vi "sequencerCore.vi"   [LabVIEW 2014]
uses:
  sequencerState.ctl
  Controls/heinzingerSelect.ctl
  <vilib>/rvi/Emulation/niFpgaGetClockAttributes.vi
  <vilib>/rvi/Emulation/niFpgaSctlEmulationGetInTimedLoop.vi
  <vilib>/rvi/Emulation/niFpgaEmulationReportErrorSimple.vi
  <vilib>/rvi/Emulation/niFpgaCriticalErrorInLSC.vi
types:
  T1 = typedef "sequencerState.ctl" = enum16{"init", "idle", "writeGlobVars", "measureOffset", "measureTrack", "measComplete", "error"}
  T2 = typedef "heinzingerSelect.ctl" = enum8{"Kepco", "Heinzinger0", "Heinzinger1", "Heinzinger2"}
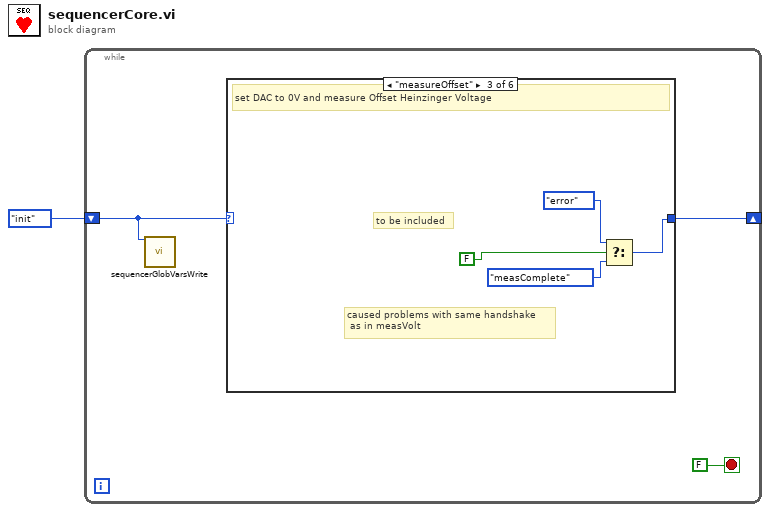
[diagram p0: block diagram]
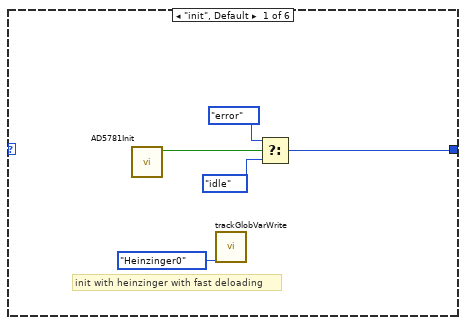
[diagram p2: hidden frame]
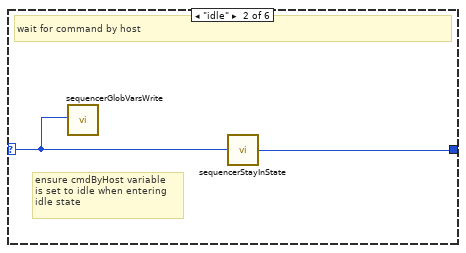
[diagram p3: hidden frame]
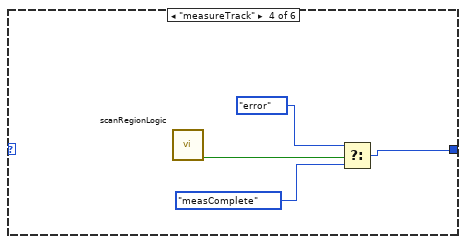
[diagram p4: hidden frame]
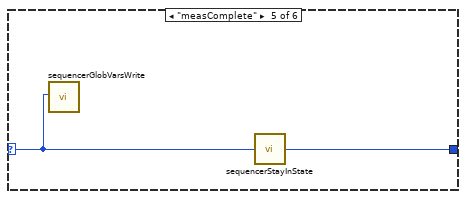
[diagram p5: hidden frame]
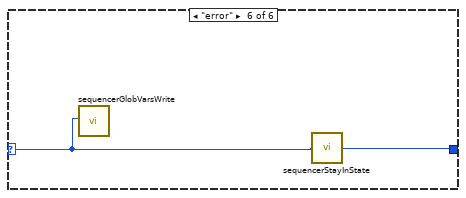
[diagram p6: hidden frame]
diagram:
  n1 = while {
    shift-right: [w2] -> _
    shift-left: sequencerState."init" ("Enum") -> [w3]
    stop <- FALSE stop-if-true
    n2 = call "sequencerGlobVarsWrite.vi"("fpgaState"=w3) -> ()  [unwired: 19 in]
    n3 = case shown="\"measureOffset\"" w3 {
      selector: w3 -> [_ w11 _ _ w21 w23]
      tunnel: [w6 w10 w15 w16 w20 w22] -> w2
      frame "init", Default {
        # "init with heinzinger with fast deloading"
        n4 = call "AD5781Init.vi"() -> ("timeOut"=w7:bool)  [unwired: 11 in]
        n5 = call "trackGlobVarWrite.vi"("heinzingerControl"=heinzingerSelect."Heinzinger0") -> ()  [unwired: 19 in]
        n6 = Select(t=sequencerState."error", s=w7, f=sequencerState."idle" ("Enum")) -> (s? t:f=w6:T1)
      }
      frame "idle" {
        # "ensure cmdByHost variable \nis set to idle when entering\nidle state"
        # "wait for command by host"
        n7 = call "sequencerGlobVarsWrite.vi"("cmdByHost"=w11) -> ()  [unwired: 19 in]
        n8 = call "sequencerStayInState.vi"("stateBefore"=w11) -> ("cmdByHost"=w10:T1)  [unwired: 4 in]
      }
      frame "measureOffset" {
        # "caused problems with same handshake\n as in measVolt"
        # "to be included"
        # "set DAC to 0V and measure Offset Heinzinger Voltage"
        n9 = Select(t=sequencerState."error" ("cmdFromHost"), s=FALSE, f=sequencerState."measComplete" ("cmdFromHost")) -> (s? t:f=w15:T1)
      }
      frame "measureTrack" {
        n10 = call "scanRegionLogic.vi"() -> ("Error"=w17:bool)  [unwired: 11 in]
        n11 = Select(t=sequencerState."error" ("Enum"), s=w17, f=sequencerState."measComplete" ("Enum")) -> (s? t:f=w16:T1)
      }
      frame "measComplete" {
        n12 = call "sequencerGlobVarsWrite.vi"("cmdByHost"=w21) -> ()  [unwired: 19 in]
        n13 = call "sequencerStayInState.vi"("stateBefore"=w21) -> ("cmdByHost"=w20:T1)  [unwired: 4 in]
      }
      frame "error" {
        n14 = call "sequencerGlobVarsWrite.vi"("cmdByHost"=w23) -> ()  [unwired: 19 in]
        n15 = call "sequencerStayInState.vi"("stateBefore"=w23) -> ("cmdByHost"=w22:T1)  [unwired: 4 in]
      }
    }
  }
